vi "Waveform Generation - Create Resources (4xI16).vi"(0 "H2T FIFO":refnum<k21>, 5 "DRAM Clock":refnum<k21>, 7 "DRAM Memory":refnum<k21>, 9 "DRAM Memory Size":u32, 11 "DRAM Ready":refnum<k21>) -> (4 "Waveform Generation Resources":T1)   [LabVIEW 2018, in "Streaming FPGA.lvlib"]
doc: "Creates the resources for the Waveform Generation.\n\nThe Waveform Generation can stream a waveform from the host through a DRAM FIFO, or it can store a waveform provided by the host in DRAM and generate it repeatedly. The waveform is read from the <B>H2T FIFO</B> Host to Target FIFO and streamed through or stored in the <B>DRAM Memory</B> memory element.\n\nThis VI must be placed on the block diagram outside of any SCTLs.\n<B>H2T FIFO</B> is the Host to Target FIFO from which the waveform samples are read, this FIFO should be configured to use I16 data type and 16 elements per read operation.\n<B>DRAM Clock</B> is the clock used by the DRAM memory interface.\nThe <B>DRAM Memory</B> memory resource must use DRAM implementation and the data type must be the type provided by the <B>Data Type (B256).ctl</B> (array of 256 booleans).\nThe <B>DRAM Memory Size</B> must be the requested number of elements parameter of the <B>DRAM Memory</B> memory resource.\n<B>DRAM Ready</B> must be an FPGA Register using the boolean data type, and this register must be set to true when the DRAM is ready.\n\nThe Waveform Generation requires the <B>Waveform Generation - Process.vi</B> to be placed on the block diagram outside of any SCTLs, and to be connected to the <B>Waveform Generation Resources</B> output of this VI.\n\nUse the <B>Waveform Generation - Read.vi</B> to control the Waveform Generation and to read the waveform samples. This VI should be placed in an SCTL (it is not necessary to clock the SCTL by the <B>DRAM Clock</B>), and needs to be connected to the <B>Waveform Generation Resources</B> output of this VI."
uses:
  Streaming FPGA.lvlib
  Waveform Generation Resources (4xI16).ctl
  Target-Scoped FIFO (4xI16) Resource.ctl
  <vilib>/rvi/DataTransferAndStorage/Container/Common/niFpgaContainerGetUniqueNameForEmu.vi
  <vilib>/rvi/DataTransferAndStorage/Container/Common/niFpgaContainerSetEmuInfo.vi
  <vilib>/rvi/eio/common/nirviEmuReportErrorAndStop.vi
  <vilib>/rvi/LocalResourceManager/LocalResourceManager.xnode
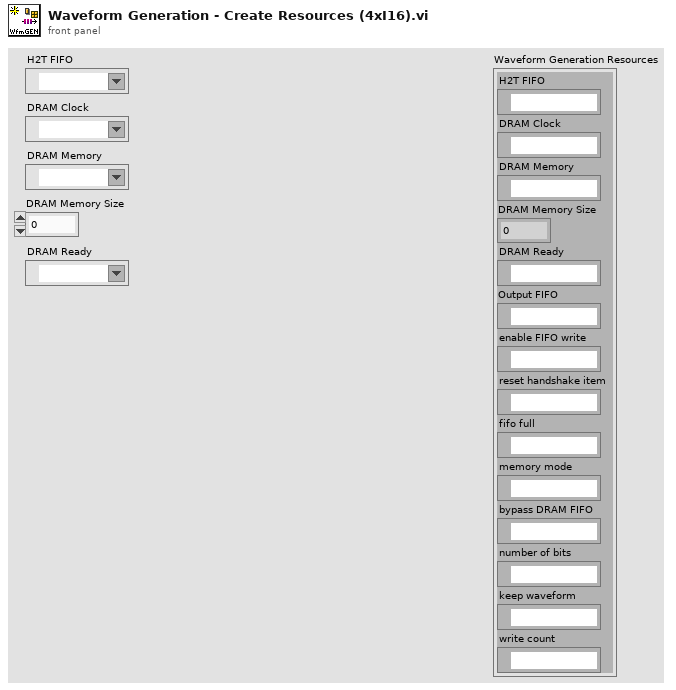
[diagram p1: front panel]
types:
  T1 = typedef "Streaming FPGA.lvlib/Waveform Generation Resources (4xI16).ctl" = cluster{"H2T FIFO":refnum<k21>, "DRAM Clock":refnum<k21>, "DRAM Memory":refnum<k21>, "DRAM Memory Size":u32, "DRAM Ready":refnum<k21>, "Output FIFO":T2, "enable FIFO write":refnum<k21>, "reset handshake item":refnum<k21>, "fifo full":refnum<k21>, "memory mode":refnum<k21>, "bypass DRAM FIFO":refnum<k21>, "number of bits":refnum<k21>, "keep waveform":refnum<k21>, "write count":refnum<k21>}
  T2 = typedef "Streaming FPGA.lvlib/Target-Scoped FIFO (4xI16) Resource.ctl" = refnum<k21>
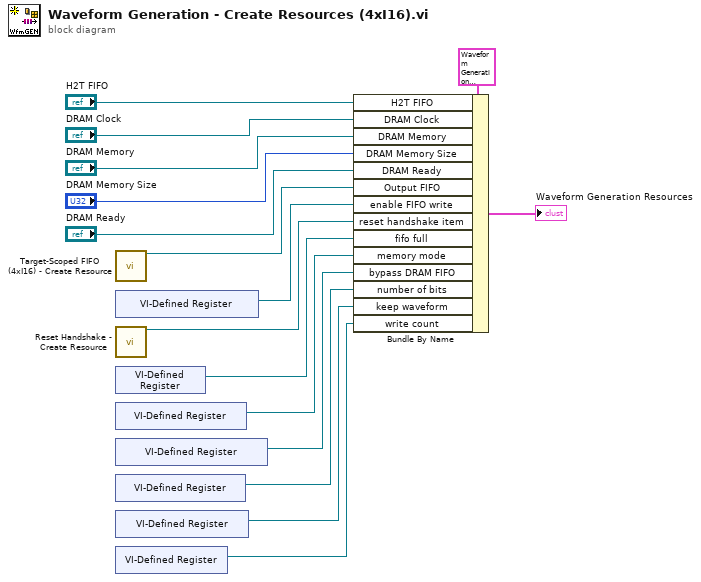
[diagram p0: block diagram]
diagram:
  n1 = call "Target-Scoped FIFO (4xI16) - Create Resource.vi"() -> ("Target-Scoped FIFO (4xI16)"=w14:T2)  [unwired: 15 in]
  n2 = xnode "VI-Defined Register"() -> ("Register Out"=w1:refnum<k21>)
  n3 = call "Reset Handshake - Create Resource.vi"() -> ("reset handshake item"=w13:refnum<k21>)  [unwired: 15 in]
  n4 = xnode "VI-Defined Register"() -> ("Register Out"=w7:refnum<k21>)
  n5 = xnode "VI-Defined Register"() -> ("Register Out"=w6:refnum<k21>)
  n6 = xnode "VI-Defined Register"() -> ("Register Out"=w5:refnum<k21>)
  n7 = xnode "VI-Defined Register"() -> ("Register Out"=w4:refnum<k21>)
  n8 = xnode "VI-Defined Register"() -> ("Register Out"=w3:refnum<k21>)
  n9 = xnode "VI-Defined Register"() -> ("Register Out"=w2:refnum<k21>)
  n10 = Bundle By Name(cluster=T1 {"H2T FIFO"="", "DRAM Clock"="", "DRAM Memory"="", "DRAM Memory Size"=0, "DRAM Ready"="", "Output FIFO"="", "enable FIFO write"="", "reset handshake item"="", "fifo full"="", "memory mode"="", "bypass DRAM FIFO"="", "number of bits"="", "keep waveform"="", "write count"=""} ("Waveform Generator Resources"), "H2T FIFO"="H2T FIFO", "DRAM Clock"="DRAM Clock", "DRAM Memory"="DRAM Memory", "DRAM Memory Size"="DRAM Memory Size", "DRAM Ready"="DRAM Ready", "Output FIFO"=w14, "enable FIFO write"=w1, "reset handshake item"=w13, "fifo full"=w7, "memory mode"=w6, "bypass DRAM FIFO"=w5, "number of bits"=w4, "keep waveform"=w3, "write count"=w2) -> (→"Waveform Generation Resources":T1)
